vi "LEP_RV_CalcOptimalHeapSize.vi"(2 "error in (no error)":errorcluster, 3 "eval mode?":bool, 4 "heap size":i32, 5 "memory regions":T1(array[cluster])) -> (0 "error out":errorcluster, 1 "optimal heap size":u32)   [LabVIEW 2011]
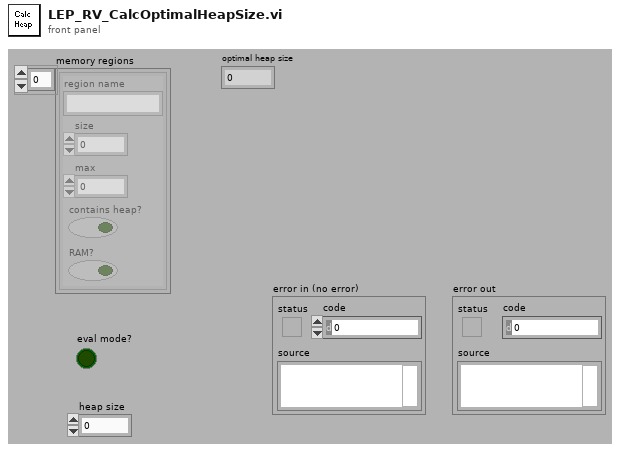
[diagram p1: front panel]
types:
  T1 = cluster{"region name":string, "size":u32, "max":u32, "contains heap?":bool, "RAM?":bool}[]
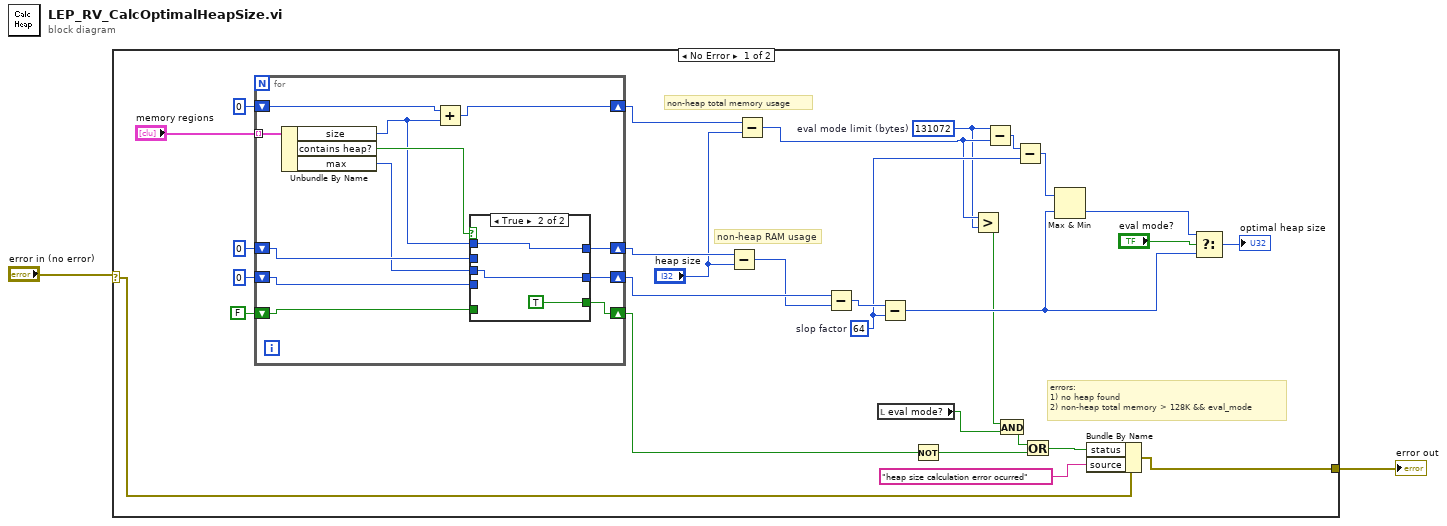
[diagram p0: block diagram]
diagram:
  n1 = case shown="No Error" "error in (no error)" {
    selector: "error in (no error)" -> [w9 w50]
    tunnel: [w6 w50] -> w1
    frame No Error {
      w12 = u32 131072  # eval mode limit (bytes)
      w19 = u32 64  # slop factor
      # "errors:\n1) no heap found\n2) non-heap total memory > 128K && eval_mode"
      # "non-heap total memory usage"
      # "non-heap RAM usage"
      n2 = for {
        tunnel: "memory regions" -> [w43] mode=indexing
        shift-right: [w41] -> w22
        shift-left: u32 0 -> [w42]
        shift-right: [w39] -> w26
        shift-left: u32 0 ("size") -> [w37]
        shift-right: [w38] -> w25
        shift-left: u32 0 ("max") -> [w36]
        shift-right: [w34] -> w10
        shift-left: FALSE -> [w35]
        n3 = Unbundle By Name(w43) -> ("size"=w33:u32, "contains heap?"=w40:bool, "max"=w32:u32)
        n4 = Add(x=w42, y=w33) -> (x+y=w41:u32)
        n5 = case shown="True" w40 {
          tunnel: [w46 w49] -> w39
          tunnel: w33 -> [_ w49]
          tunnel: w32 -> [_ w48]
          tunnel: [w45 w48] -> w38
          tunnel: w37 -> [w46 _]
          tunnel: w36 -> [w45 _]
          tunnel: w35 -> [w44 _]
          tunnel: [w44 TRUE] -> w34
          frame False {
          }
          frame True {
          }
        }
      }
      n6 = Subtract(x=w26, y="heap size") -> (x-y=w24:u32)
      n7 = Subtract(x=w22, y="heap size") -> (x-y=w13:u32)
      n8 = Subtract(x=w25, y=w24) -> (x-y=w23:u32)
      n9 = local read "eval mode?"() -> (w5:bool)
      n10 = Subtract(x=w23, y=w19) -> (x-y=w15:u32)
      n11 = Not(x=w10) -> (.not. x?=w11:bool)
      n12 = Greater?(x=w13, y=w12) -> (0:w4:bool)
      n13 = Subtract(x=w12, y=w13) -> (x-y=w20:u32)
      n14 = And(x=w4, y=w5) -> (x .and. y?=w3:bool)
      n15 = Subtract(x=w20, y=w19) -> (x-y=w18:u32)
      n16 = Or(x=w3, y=w11) -> (x .or. y?=w8:bool)
      n17 = Max & Min(x=w18, y=w15) -> (min(x,y)=w16:u32)  [unwired: 1 out]
      n18 = Bundle By Name(cluster=w9, "status"=w8, "source"="heap size calculation error ocurred") -> (w6:errorcluster)
      n19 = Select(t=w16, s="eval mode?", f=w15) -> (s? t:f=→"optimal heap size":u32)
    }
    frame Error {
    }
  }
  "error out" <- w1
